vi "Check if Message Exists.vi"(7 "Target":refnum<vi>, 8 "error in (no error)":errorcluster, 10 "Method Name":string, 11 "Actor":refnum<vi>) -> (0 "error out":errorcluster, 2 "Message Class Exists?":bool, 3 "Message Path":path)   [LabVIEW 2020, in "Message Maker.lvlib"]
uses:
  Message Maker.lvlib
  <vilib>/ErrorRing/Error Ring.xnode
  <vilib>/Utility/error.llb/Error Cluster From Error Code.vi
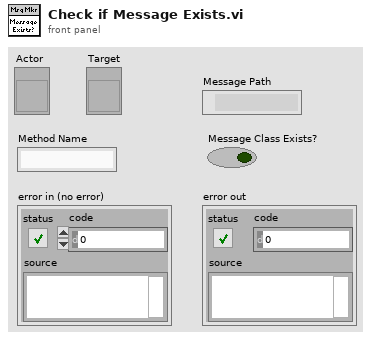
[diagram p1: front panel]
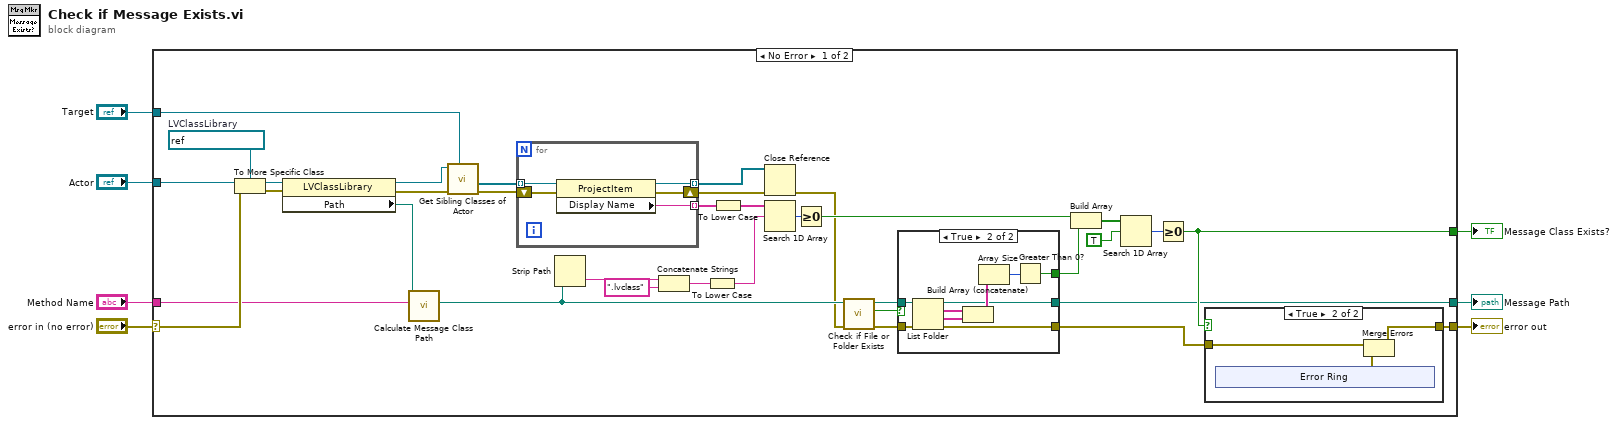
[diagram p0: block diagram]
diagram:
  n1 = case shown="No Error" "error in (no error)" {
    selector: "error in (no error)" -> [w33 w68]
    tunnel: "Method Name" -> [w32 _]
    tunnel: "Actor" -> [w42 _]
    tunnel: [w10 _] -> w5
    tunnel: [w14 w68] -> w4
    tunnel: [w15 _] -> w3
    tunnel: "Target" -> [w28 _]
    frame No Error {
      w40 = refnum<vi> refnum  # LVClassLibrary
      n2 = To More Specific Class(target class=w40, reference=w42, error in=w33) -> (specific class reference=w41:refnum<vi>, error out=w36:errorcluster)
      n3 = property class="LVClassLibrary"(reference=w41, error in=w36) -> (reference out=w18:refnum<vi>, error out=w31:errorcluster, "Path"=w39:path)
      n4 = call "Calculate Message Class Path.vi"("Method VI Name"=w32, "Actor Class Path"=w39) -> ("Message Class Path"=w35:path)  [unwired: 9 in]
      n5 = call "Get Sibling Classes of Actor.vi"("Target"=w28, "error in (no error)"=w31, "Actor"=w18) -> ("error out"=w19:errorcluster, "Sibling Classes"=w24:refnum<vi>[])  [unwired: 7 in]
      n6 = for {
        tunnel: w24 -> [w67] mode=indexing
        shift-right: [w65] -> w38
        shift-left: w19 -> [w66]
        tunnel: [w64] -> w37 mode=indexing
        tunnel: [w63] -> w29 mode=indexing
        n7 = property class="ProjectItem"(reference=w67, error in=w66) -> (reference out=w64:refnum<vi>, error out=w65:errorcluster, "Display Name"=w63:string)
      }
      n8 = Strip Path(path=w35) -> (name=w30:string)  [unwired: 1 out]
      n9 = Concatenate Strings(w30, ".lvclass" ("string")) -> (w27:string)
      n10 = To Lower Case(string=w27) -> (all lower case string=w16:string)
      n11 = To Lower Case(string=w29) -> (all lower case string=w17:string[])
      n12 = Close Reference(reference=w37, error in (no error)=w38) -> (error out=w23:errorcluster)
      n13 = Search 1D Array(1D array=w17, element=w16) -> (index of element=w34:i32)  [unwired: 1 in]
      n14 = Greater Or Equal To 0?(x=w34) -> (x >= 0?=w25:bool)
      n15 = call <vilib>:"Check if File or Folder Exists.vi"("error in (no error)"=w23, "path"=w35) -> ("error out"=w13:errorcluster, "file or folder exists?"=w11:bool, "dup path"=w12:path)  [unwired: 7 in]
      n16 = case shown="True" w11 {
        tunnel: w13 -> [w44 w53]
        tunnel: w12 -> [w43 w52]
        tunnel: [w44 w49] -> w9
        tunnel: [w43 w47] -> w10
        tunnel: [_ w45] -> w8
        frame False {
        }
        frame True {
          n17 = List Folder(path=w52, error in=w53) -> (path out=w47:path, filenames=w50:string[], folder names=w51:string[], error out=w49:errorcluster)  [unwired: 2 in]
          n18 = Build Array (concatenate)(w50, w51) -> (w48:string[])
          n19 = Array Size(array=w48) -> (size(s)=w46:i32)
          n20 = Greater Than 0?(x=w46) -> (x > 0?=w45:bool)
        }
      }
      n21 = Build Array(w25, w8) -> (w22:bool[])
      n22 = Search 1D Array(1D array=w22, element=TRUE) -> (index of element=w21:i32)  [unwired: 1 in]
      n23 = Greater Or Equal To 0?(x=w21) -> (x >= 0?=w15:bool)
      n24 = case shown="True" w15 {
        tunnel: w9 -> [w54 w57]
        tunnel: [w54 w55] -> w14
        frame False {
        }
        frame True {
          n25 = xnode "Error Ring"() -> ("error out"=w56:errorcluster)
          n26 = Merge Errors(w57, w56) -> (w55:errorcluster)
        }
      }
    }
    frame Error {
    }
  }
  "Message Class Exists?" <- w3
  "error out" <- w4
  "Message Path" <- w5
